vi "Server.vi"() -> ()   [LabVIEW 2020]
uses:
  <vilib>/DatastreamGrpc/DatastreamGrpc.lvlib
panel:
  out "time string":string
  in  "stop":bool
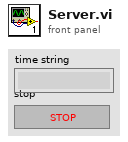
[diagram p1: front panel]
types:
  T1 = typedef "DatastreamGrpc.lvlib/ServerRef.ctl" = cluster{"id":u64}
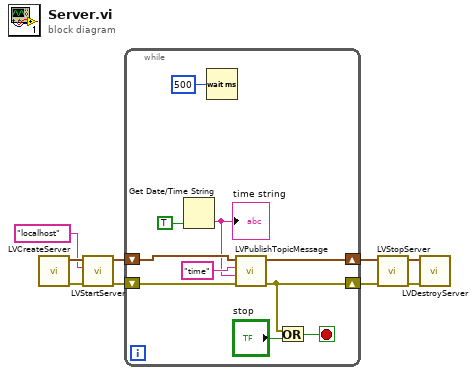
[diagram p0: block diagram]
diagram:
  n1 = call <vilib>:"LVCreateServer.vi"() -> ("error out"=w8:errorcluster, "ServerRef out"=w9:T1)  [unwired: 10 in]
  n2 = call <vilib>:"LVStartServer.vi"("error in (no error)"=w8, "address"="localhost", "ServerRef in"=w9) -> ("error out"=w3:errorcluster, "ServerRef out"=w4:T1)  [unwired: 7 in]
  n3 = while {
    shift-right: [w17] -> w1
    shift-left: w4 -> [w19]
    shift-right: [w11] -> w2
    shift-left: w3 -> [w18]
    stop <- w12 stop-if-true
    n4 = Get Date/Time String(want seconds? (F)=TRUE) -> (time string=w15:string)  [unwired: 2 in, 1 out]
    "time string" <- w15
    n5 = Wait (ms)(milliseconds to wait=u32 500) -> ()  [unwired: 1 out]
    n6 = call <vilib>:"LVPublishTopicMessage.vi"("error in (no error)"=w18, "MessageData"=w15, "TopicName"="time", "ServerRef in"=w19) -> ("error out"=w11:errorcluster, "ServerRef out"=w17:T1)  [unwired: 6 in]
    n7 = Or(x=w11, y="stop") -> (x .or. y?=w12:bool)
  }
  n8 = call <vilib>:"LVStopServer.vi"("error in (no error)"=w2, "ServerRef in"=w1) -> ("error out"=w6:errorcluster, "ServerRef out"=w5:T1)  [unwired: 8 in]
  n9 = call <vilib>:"LVDestroyServer.vi"("error in (no error)"=w6, "ServerRef in"=w5) -> ()  [unwired: 9 in, 1 out]
